vi "All_ThingsSummer2020.vi"   [LabVIEW 2020]
uses:
  Subs/RestAPI.ctl
  Subs/ColorText/ColorGlobals.vi
  Subs/SystemLink/SL_Subs/SystemLink_Write_String.vi
  Subs/JSON_Formats.vi
types:
  T1 = typedef "RestAPI.ctl" = cluster{"headers 2":string, "headers":string, "body":string}
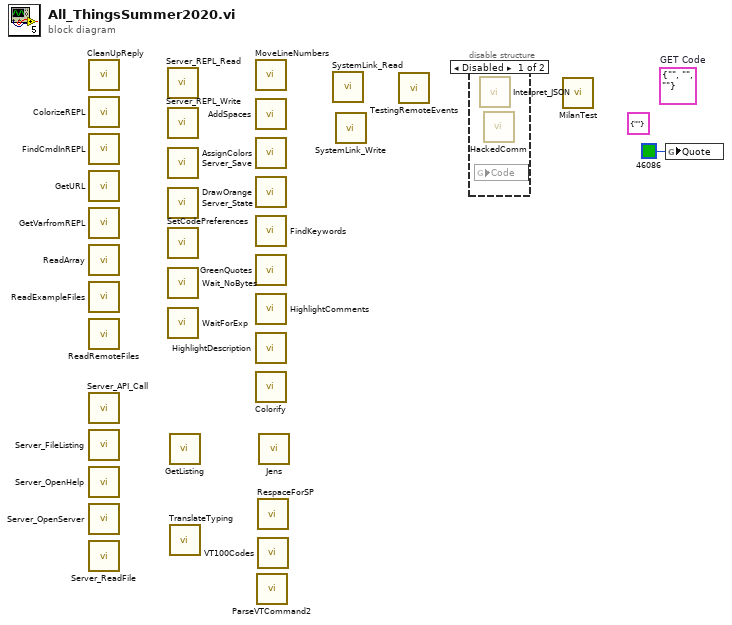
[diagram p0: block diagram]
diagram:
  (unwired) cluster{"Code":string} {"Code"=""} ("Code")
  (unwired) T1 {"headers 2"="", "headers"="", "body"=""}  # GET Code
  n1 = call "CleanUpReply.vi"() -> ()  [unwired: 11 in, 1 out]
  n2 = call "ColorizeREPL.vi"() -> ()  [unwired: 10 in, 1 out]
  n3 = call "FindCmdInREPL.vi"() -> ()  [unwired: 11 in, 1 out]
  n4 = call "GetURL.vi"() -> ()  [unwired: 8 in, 4 out]
  n5 = call "GetVarfromREPL.vi"() -> ()  [unwired: 10 in, 2 out]
  n6 = call "ReadArray.vi"() -> ()  [unwired: 11 in, 1 out]
  n7 = call "ReadExampleFiles.vi"() -> ()  [unwired: 12 in]
  n8 = call "ReadRemoteFiles.vi"() -> ()  [unwired: 12 in]
  n9 = call "Server_API_Call.vi"() -> ()  [unwired: 8 in, 4 out]
  n10 = call "Server_FileListing.vi"() -> ()  [unwired: 8 in, 4 out]
  n11 = call "Server_OpenHelp.vi"() -> ()  [unwired: 11 in, 1 out]
  n12 = call "Server_OpenServer.vi"() -> ()  [unwired: 11 in, 1 out]
  n13 = call "Server_ReadFile.vi"() -> ()  [unwired: 10 in, 2 out]
  n14 = call "Server_REPL_Read.vi"() -> ()  [unwired: 9 in, 3 out]
  n15 = call "Server_REPL_Write.vi"() -> ()  [unwired: 11 in, 1 out]
  n16 = call "Server_Save.vi"() -> ()  [unwired: 11 in, 1 out]
  n17 = call "Server_State.vi"() -> ()  [unwired: 9 in, 3 out]
  n18 = call "SetCodePreferences.vi"() -> ()  [unwired: 12 in]
  n19 = call "Wait_NoBytes.vi"() -> ()  [unwired: 10 in, 2 out]
  n20 = call "WaitForExp.vi"() -> ()  [unwired: 10 in, 2 out]
  n21 = call "GetListing.vi"() -> ()  [unwired: 9 in, 3 out]
  n22 = call "TranslateTyping.vi"() -> ()  [unwired: 11 in, 1 out]
  n23 = call "MoveLineNumbers.vi"() -> ()  [unwired: 12 in]
  n24 = call "AddSpaces.vi"() -> ()  [unwired: 10 in, 2 out]
  n25 = call "AssignColors.vi"() -> ()  [unwired: 11 in, 1 out]
  n26 = call "DrawOrange.vi"() -> ()  [unwired: 11 in, 1 out]
  n27 = call "FindKeywords.vi"() -> ()  [unwired: 11 in, 1 out]
  n28 = call "GreenQuotes.vi"() -> ()  [unwired: 11 in, 1 out]
  n29 = call "HighlightComments.vi"() -> ()  [unwired: 11 in, 1 out]
  n30 = call "HighlightDescription.vi"() -> ()  [unwired: 11 in, 1 out]
  n31 = call "Colorify.vi"() -> ()  [unwired: 12 in]
  n32 = call "ParseVTCommand2.vi"() -> ()  [unwired: 7 in, 5 out]
  n33 = call "RespaceForSP.vi"() -> ()  [unwired: 11 in, 1 out]
  n34 = call "VT100Codes.vi"() -> ()  [unwired: 11 in, 1 out]
  n35 = call "Jens.vi"() -> ()  [unwired: 12 in]
  n36 = call "SystemLink_Read.vi"() -> ()  [unwired: 9 in, 3 out]
  n37 = call-poly "SystemLink_Write.vi"() -> ()  [unwired: 12 in]
  n38 = call "TestingRemoteEvents.vi"() -> ()  [unwired: 12 in]
  n39 = disable-structure shown="Disabled" {
    frame Disabled {
      n40 = global read "JSON_Formats.vi" "Code"() -> ()  [unwired: 1 in]
      n41 = call "Interpret_JSON.vi"() -> ()  [unwired: 9 in, 3 out]
      n42 = call "HackedComm.vi"() -> ()  [unwired: 10 in, 2 out]
    }
    frame Enabled {
    }
  }
  n43 = call "MilanTest.vi"() -> ()  [unwired: 12 in]
  n44 = global write "ColorGlobals.vi" "Quote"(u32 46086 ("Quote")) -> ()
